vi "ReadBase.vi"(8 "error in (no error)":errorcluster, 10 "Request Number of Message":i32, 11 "GenericCanAdapterClass in":refnum<class "GenericCanAdapterClass.lvclass">) -> (0 "error out":errorcluster, 2 "Messages":T1[](array[typedef]) {"Data" format="%02x"; "Arbitration Id" format="%03x"}, 3 "GenericCanAdapterClass out":refnum<class "GenericCanAdapterClass.lvclass">)   [LabVIEW 2011, in "GenericCanAdapterClass.lvclass"]
uses:
  GenericCanAdapterClass.lvclass
  National Instruments USB-8473 Adapter/MessageType.ctl
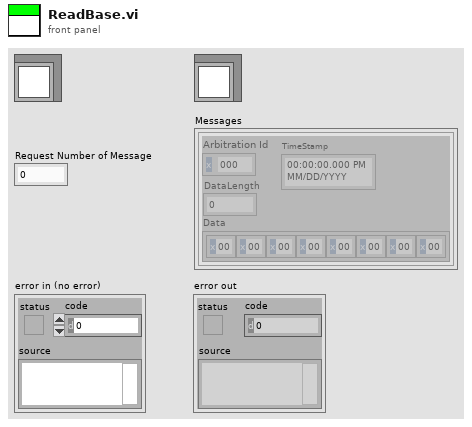
[diagram p1: front panel]
types:
  T1 = typedef "GenericCanAdapterClass.lvclass/MessageType.ctl" = cluster{"Arbitration Id":u32, "Data":u8[], "DataLength":u16, "TimeStamp":timestamp}
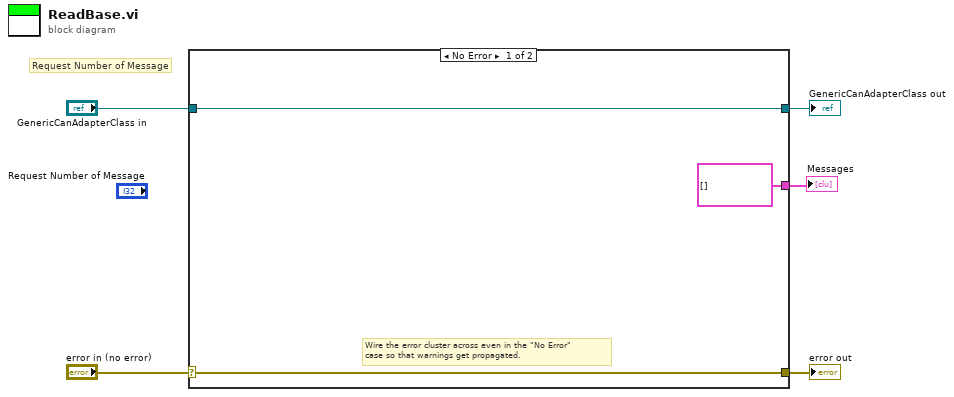
[diagram p0: block diagram]
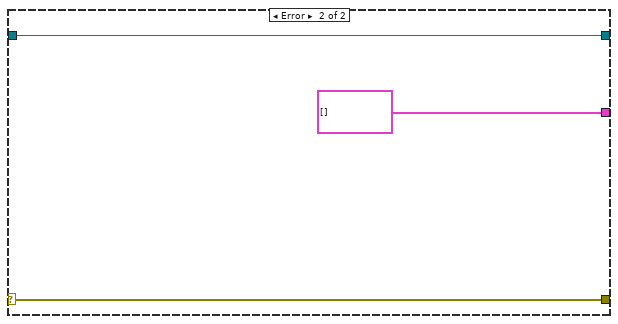
[diagram p2: hidden frame]
diagram:
  # "Request Number of Message"
  n1 = case shown="No Error" "error in (no error)" {
    selector: "error in (no error)" -> [w7 w11]
    tunnel: [w7 w11] -> w4
    tunnel: [w8 w10] -> w2
    tunnel: "GenericCanAdapterClass in" -> [w8 w10]
    tunnel: [T1[] [] T1[] []] -> w1
    frame No Error {
      # "Wire the error cluster across even in the \"No Error\"\ncase so that warnings get propagated."
    }
    frame Error {
    }
  }
  "error out" <- w4
  "GenericCanAdapterClass out" <- w2
  "Messages" <- w1
